vi "Array Subset.vi"() -> ()   [LabVIEW 2016]
panel:
  out "Array 2":dbl[](array[numeric])
  in  "Length":dbl
  in  "Index":dbl
  in  "Array":dbl[](array[numeric])
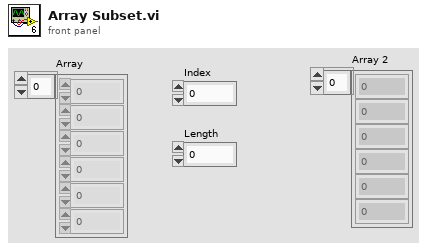
[diagram p1: front panel]
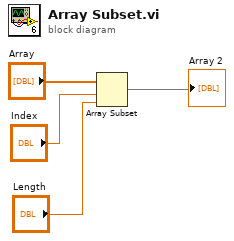
[diagram p0: block diagram]
diagram:
  n1 = Array Subset(array="Array", index="Index", length="Length") -> (→"Array 2":dbl[])
